vi "ObtainQueue.vi"(5 "Max Queue Size (-1, Unlimited)":i32=-1, 7 "Create If Not Found? (T)":bool=TRUE, 8 "error in (no error)":errorcluster, 11 "Queue Name":string) -> (0 "error out":errorcluster, 1 "Created New?":bool, 3 "MessageQueue out":refnum<class "MessageQueue.lvclass">)   [LabVIEW 2017, in "LapDog.Messaging.v3.lvlib" / "MessageQueue.lvclass"]
doc: "Returns a fully configured MessageQueue object.\n\nMessageQueue's behavior is very similar to native Labview queues, with the exception that the queue can only transport Message objects instead of arbitrary data types."
uses:
  MessageQueue.lvclass
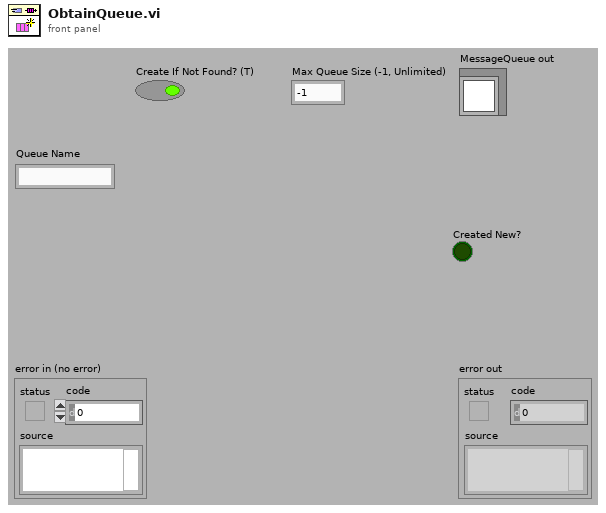
[diagram p1: front panel]
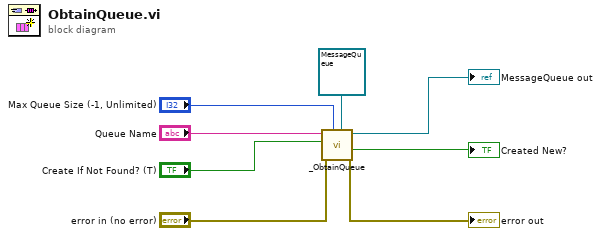
[diagram p0: block diagram]
diagram:
  n1 = call "_ObtainQueue.vi"("MessageQueue Type"=refnum<class "MessageQueue.lvclass"> refnum ("MessageQueue in"), "Max Queue Size (-1, unlimited)"="Max Queue Size (-1, Unlimited)", "error in (no error)"="error in (no error)", "Create if Not Found? (T)"="Create If Not Found? (T)", "Queue Name"="Queue Name") -> ("error out"=→"error out":errorcluster, "Created New?"=→"Created New?":bool, "MessageQueue out"=→"MessageQueue out":refnum<class "MessageQueue.lvclass">)  [unwired: 4 in]
